vi "nanocal -- nuclear schottky fit V7.vi"() -> ()   [LabVIEW 2021] (continued)
  in  ":sweep is ON":bool
  in  "win":T16={"cen (Hz)"=23772.179970264126, "win (Hz)"=4484.832860239923, "left (Hz)"=21529.763540144166, "right (Hz)"=26014.596400384085}
  in  "cursor window":T17={"left"=20184.313682072192, "right "=24669.14654231211, "center"=22426.730112192152, "window"=4484.832860239923, "cursors"=[0, 1, 2], "relative"=0, "absolute"=0, "fixed vertical offset"=0.0, "vertical offset"=0.0, "skew"=0.0, "default window frac"=0.1, "kind"=enum."symmetric", "skew.left"=0.5, "skew.right"=0.5, "Plot ref"=refnum, "wing order"=enum."forw"}
  out "color data":cluster{"Array":dbl[], "Array":dbl[]}[](array[cluster])=[{"Array"=[0.12, 0.148, 0.15, 0.17, 0.2, 0.25, 0.3, 0.36, 0.42, 0.52, 0.62, 0.82, 1.12, 1.7, 1.9, 3.1, 5.7], "Array"=[0.62728998582, 0.2730109012575849, 0.4360358231158382, 0.31273882707493267, 0.21185679953244455, 0.14497429295634315, 0.10320507255338958, 0.06738649827292763, 0.022507492936216303, 0.021849716434935364, 0.021729475893381252, 0.0198519726342436, 0.016283381951146165, 0.01886089700009046, 0.017534515105553365, 0.01657901647493233, 0.017491792324152208]}, {"Array"=[0.12, 0.148, 0.15, 0.17, 0.2, 0.25, 0.3, 0.36, 0.42, 0.52, 0.62, 0.82, 1.12, 1.7, 1.9, 3.1, 5.7], "Array"=[0.23974349678, 0.07091543775458298, 0.13629832485566626, 0.15316677568416495, 0.17371303124805412, 0.27815367910908206, 0.4568771678095196, 0.03375938315839582, 0.03387143424300576, 0.033883152649051125, 0.03390178634313435, 0.03384656153160249, 0.03390452446017073, 0.03378369231014688, 0.02323861783817173, 0.029207680038740087, 0.02587551529326107]}, {"Array"=[0.12, 0.148, 0.15, 0.17, 0.2, 0.25, 0.3, 0.36, 0.42, 0.52, 0.62, 0.82, 1.12, 1.7, 1.9, 3.1, 5.7], "Array"=[0.076926495749, 0.13557684408337248, 0.03542880244691447, 0.02942840377205427, 0.02504707721851352, 0.020087180736490247, 0.018190810679879554, 0.0163524675075112, 0.016835987172777216, 0.01819702773822382, 0.020153498516221252, 0.023547995635674095, 0.031661688913314306, 0.03349591654527996, 0.014265591932458873, 0.009191722708188048, 0.005854448603805341]}, {"Array"=[0.12, 0.148, 0.15, 0.17, 0.2, 0.25, 0.3, 0.36, 0.42, 0.52, 0.62, 0.82, 1.12, 1.7, 1.9, 3.1, 5.7], "Array"=[0.159415903746, 0.04012911681217574, 0.042141009445427945, 0.032059842594624494, 0.02279985029361622, 0.018878235168909133, 0.020353539568818982, 5.5602042137039274e-05, 0.00021346840235837033, 0.00021340250099372794, 0.00021321792059620005, 0.00027413175252649695, 0.0002745370162211529, 0.0004261574975821111, 0.000383027800546881, 0.0002822141564676873, 0.00033678261197217014]}, {"Array"=[0.12, 0.148, 0.15, 0.17, 0.2, 0.25, 0.3, 0.36, 0.42, 0.52, 0.62, 0.82, 1.12, 1.7, 1.9, 3.1, 5.7], "Array"=[0.000763641667, 0.0009923872987074498, 0.0008634344957269274, 0.000966119229084584, 0.0011194877919145127, 0.0013606502621125451, 0.0015326336783234693, 0.002052818741953473, 0.0017781658353584764, 0.001801850307392029, 0.0018089734240976446, 0.002984103948241005, 0.003250738484609814, 0.0031602960429135524, 0.002949269667352954, 0.002421267656945163, 0.002022629565026247]}, {"Array"=[0.12, 0.148, 0.15, 0.17, 0.2, 0.25, 0.3, 0.36, 0.42, 0.52, 0.62, 0.82, 1.12, 1.7, 1.9, 3.1, 5.7], "Array"=[4.35e-10, 6.439381253023805e-10, 6.308810838918409e-10, 7.625114350763984e-10, 8.195852207774218e-10, 1.2510608054547487e-09, 1.5572561005318226e-09, 2.053450896656566e-09, 2.479707154238972e-09, 3.1313474594286157e-09, 3.806148532350378e-09, 5.213755545903577e-09, 7.2628137959888106e-09, 1.1406421503525573e-08, 1.2895431292182517e-08, 2.227660928974633e-08, 5.4777678949124484e-08]}, {"Array"=[0.12, 0.148, 0.15, 0.17, 0.2, 0.25, 0.3, 0.36, 0.42, 0.52, 0.62, 0.82, 1.12, 1.7, 1.9, 3.1, 5.7], "Array"=[0.245568364347, 0.0645900574929368, 0.08004705050622966, 0.19487148720579237, 0.03351434142711687, 0.02184431417017586, 0.032347659490051216, 0.002480419109659059, 0.007814821925534395, 0.00520013588180238, 0.006296094438005391, 0.001908169809423058, 0.002257620140211018, 0.008605835968785608, 0.0024989962580555026, 0.003215464238537897, 0.003570816055454911]}, {"Array"=[0.12, 0.148, 0.15, 0.17, 0.2, 0.25, 0.3, 0.36, 0.42, 0.52, 0.62, 0.82, 1.12, 1.7, 1.9, 3.1, 5.7], "Array"=[0.022170590915, 0.01641248298202389, 0.002312030386804106, 0.0014819318949486784, 0.00035662888776441895, 0.00015894172062156444, 0.00010225804136915292, 0.0001282920284827463, 0.0003857404741353476, 0.00019678175234393364, 0.0002692480741424916, 0.00013393087590862188, 0.00016283980709594313, 0.00045778261364612133, 0.0003120318371061343, 8.8801730217525e-05, 7.291236500401702e-05]}, {"Array"=[0.12, 0.148, 0.15, 0.17, 0.2, 0.25, 0.3, 0.36, 0.42, 0.52, 0.62, 0.82, 1.12, 1.7, 1.9, 3.1, 5.7], "Array"=[0.126655465898, 0.016122106455977173, 0.019370507574418105, 0.032515587695104, 0.003953255270019443, 0.0013746091281296251, 0.0011727018719404464, 1.3396144617265272e-06, 1.8309382419984372e-05, 1.6694885155659994e-05, 1.6264646942714422e-05, 2.638451785235589e-06, 9.699549898748168e-06, 7.027190427402306e-05, 9.499625775806485e-06, 1.529926658584193e-05, 2.3576375004937536e-05]}]
  out "R(ω) fit out":cdb[](array[numeric])
  in  "parameter map":map{T2, dbl}(c390)
  out "filesnames lookup":map{i32, string}(c390)={0="IDS0183_210310_RAW_cal__sam_", 1="IDS0311_210901_RAW_cal__sam_", 2="IDS0359_210907_RAW_cal__sam_", 3="IDS0412_220525_RAW_cal__sam_", 4="IDS0431_220527_RAW_cal__sam_", 5="IDS0442_220528_RAW_cal__sam_", 6="IDS0464_220530_RAW_cal__sam_", 7="IDS0486_220602_RAW_cal__sam_", 8="IDS0336_210904_RAW_cal__sam_", 9="IDS0346_210904_RAW_cal__sam_", 10="IDS0378_210909_RAW_cal__sam_", 11="IDS0158_210310_RAW_cal__sam_", 12="IDS0300_210427_RAW_cal__sam_", 13="IDS0184_210310_RAW_cal__sam_", 14="IDS0210_210310_RAW_cal__sam_", 15="IDS0379_210909_RAW_cal__sam_", 16="IDS0360_210907_RAW_cal__sam_", 17="IDS0411_220525_RAW_cal__sam_", 18="IDS0427_220526_RAW_cal__sam_", 19="IDS0443_220528_RAW_cal__sam_", 20="IDS0463_220530_RAW_cal__sam_", 21="IDS0487_220602_RAW_cal__sam_", 22="IDS0310_210901_RAW_cal__sam_", 23="IDS0337_210904_RAW_cal__sam_", 24="IDS0347_210906_RAW_cal__sam_", 25="IDS0305_210831_RAW_cal__sam_", 26="IDS0361_210908_RAW_cal__sam_", 27="IDS0380_210909_RAW_cal__sam_", 28="IDS0159_210310_RAW_cal__sam_", 29="IDS0304_210831_RAW_cal__sam_", 30="IDS0312_210901_RAW_cal__sam_", 31="IDS0338_210904_RAW_cal__sam_", 32="IDS0410_220525_RAW_cal__sam_", 33="IDS0432_220527_RAW_cal__sam_", 34="IDS0444_220528_RAW_cal__sam_", 35="IDS0462_220530_RAW_cal__sam_", 36="IDS0485_220601_RAW_cal__sam_", 37="IDS0348_210906_RAW_cal__sam_", 38="IDS0181_210310_RAW_cal__sam_", 39="IDS0424_220526_RAW_cal__sam_", 40="IDS0185_210310_RAW_cal__sam_", 41="IDS0208_210310_RAW_cal__sam_", 42="IDS0209_210310_RAW_cal__sam_", 43="IDS0211_210310_RAW_cal__sam_", 44="IDS0212_210310_RAW_cal__sam_", 45="IDS0213_210310_RAW_cal__sam_", 46="IDS0214_210310_RAW_cal__sam_", 47="IDS0215_210310_RAW_cal__sam_", 48="IDS0216_210310_RAW_cal__sam_", 49="IDS0217_210310_RAW_cal__sam_", 50="IDS0330_210901_RAW_cal__sam_", 51="IDS0331_210901_RAW_cal__sam_", 52="IDS0335_210904_RAW_cal__sam_", 53="IDS0362_210908_RAW_cal__sam_", 54="IDS0377_210909_RAW_cal__sam_", 55="IDS0160_210310_RAW_cal__sam_", 56="IDS0303_210831_RAW_cal__sam_", 57="IDS0313_210901_RAW_cal__sam_", 58="IDS0349_210906_RAW_cal__sam_", 59="IDS0407_220525_RAW_cal__sam_", 60="IDS0441_220527_RAW_cal__sam_", 61="IDS0458_220529_RAW_cal__sam_", 62="IDS0477_220601_RAW_cal__sam_", 63="IDS0161_210310_RAW_cal__sam_", 64="IDS0186_210310_RAW_cal__sam_", 65="IDS0302_210831_RAW_cal__sam_", 66="IDS0363_210908_RAW_cal__sam_", 67="IDS0381_210909_RAW_cal__sam_", 68="IDS0408_220525_RAW_cal__sam_", 69="IDS0425_220526_RAW_cal__sam_", 70="IDS0445_220528_RAW_cal__sam_", 71="IDS0459_220529_RAW_cal__sam_", 72="IDS0478_220601_RAW_cal__sam_", 73="IDS0314_210901_RAW_cal__sam_", 74="IDS0339_210904_RAW_cal__sam_", 75="IDS0350_210906_RAW_cal__sam_", 76="IDS0162_210310_RAW_cal__sam_", 77="IDS0187_210310_RAW_cal__sam_", 78="IDS0301_210831_RAW_cal__sam_", 79="IDS0315_210901_RAW_cal__sam_", 80="IDS0382_210909_RAW_cal__sam_", 81="IDS0409_220525_RAW_cal__sam_", 82="IDS0426_220526_RAW_cal__sam_", 83="IDS0446_220528_RAW_cal__sam_", 84="IDS0460_220529_RAW_cal__sam_", 85="IDS0479_220601_RAW_cal__sam_", 86="IDS0364_210908_RAW_cal__sam_", 87="IDS0340_210904_RAW_cal__sam_", 88="IDS0351_210906_RAW_cal__sam_", 89="IDS0163_210310_RAW_cal__sam_", 90="IDS0188_210310_RAW_cal__sam_", 91="IDS0299_210427_RAW_cal__sam_", 92="IDS0316_210901_RAW_cal__sam_", 93="IDS0341_210904_RAW_cal__sam_", 94="IDS0352_210906_RAW_cal__sam_", 95="IDS0365_210908_RAW_cal__sam_", 96="IDS0383_210910_RAW_cal__sam_", 97="IDS0413_220525_RAW_cal__sam_", 98="IDS0428_220526_RAW_cal__sam_", 99="IDS0447_220528_RAW_cal__sam_", 100="IDS0461_220529_RAW_cal__sam_", 101="IDS0480_220601_RAW_cal__sam_", 102="IDS0164_210310_RAW_cal__sam_", 103="IDS0429_220526_RAW_cal__sam_", 104="IDS0448_220528_RAW_cal__sam_", 105="IDS0481_220601_RAW_cal__sam_", 106="IDS0189_210310_RAW_cal__sam_", 107="IDS0298_210427_RAW_cal__sam_", 108="IDS0317_210901_RAW_cal__sam_", 109="IDS0366_210908_RAW_cal__sam_", 110="IDS0384_210910_RAW_cal__sam_", 111="IDS0414_220525_RAW_cal__sam_", 112="IDS0465_220530_RAW_cal__sam_", 113="IDS0342_210904_RAW_cal__sam_", 114="IDS0353_210906_RAW_cal__sam_", 115="IDS0165_210310_RAW_cal__sam_", 116="IDS0190_210310_RAW_cal__sam_", 117="IDS0430_220526_RAW_cal__sam_", 118="IDS0449_220528_RAW_cal__sam_", 119="IDS0482_220601_RAW_cal__sam_", 120="IDS0297_210427_RAW_cal__sam_", 121="IDS0318_210901_RAW_cal__sam_", 122="IDS0343_210904_RAW_cal__sam_", 123="IDS0354_210906_RAW_cal__sam_", 124="IDS0367_210908_RAW_cal__sam_", 125="IDS0385_210910_RAW_cal__sam_", 126="IDS0415_220525_RAW_cal__sam_", 127="IDS0466_220530_RAW_cal__sam_", 128="IDS0166_210310_RAW_cal__sam_", 129="IDS0191_210310_RAW_cal__sam_", 130="IDS0296_210427_RAW_cal__sam_", 131="IDS0319_210901_RAW_cal__sam_", 132="IDS0344_210904_RAW_cal__sam_", 133="IDS0433_220527_RAW_cal__sam_", 134="IDS0450_220528_RAW_cal__sam_", 135="IDS0467_220530_RAW_cal__sam_", 136="IDS0483_220601_RAW_cal__sam_", 137="IDS0368_210908_RAW_cal__sam_", 138="IDS0386_210910_RAW_cal__sam_", 139="IDS0416_220525_RAW_cal__sam_", 140="IDS0220_210310_RAW_cal__sam_", 141="IDS0167_210310_RAW_cal__sam_", 142="IDS0192_210310_RAW_cal__sam_", 143="IDS0434_220527_RAW_cal__sam_", 144="IDS0451_220528_RAW_cal__sam_", 145="IDS0468_220530_RAW_cal__sam_", 146="IDS0484_220601_RAW_cal__sam_", 147="IDS0295_210427_RAW_cal__sam_", 148="IDS0320_210901_RAW_cal__sam_", 149="IDS0355_210906_RAW_cal__sam_", 150="IDS0369_210908_RAW_cal__sam_", 151="IDS0387_210910_RAW_cal__sam_", 152="IDS0417_220525_RAW_cal__sam_", 153="IDS0168_210310_RAW_cal__sam_", 154="IDS0219_210310_RAW_cal__sam_", 155="IDS0193_210310_RAW_cal__sam_", 156="IDS0418_220525_RAW_cal__sam_", 157="IDS0435_220527_RAW_cal__sam_", 158="IDS0452_220528_RAW_cal__sam_", 159="IDS0469_220530_RAW_cal__sam_", 160="IDS0488_220602_RAW_cal__sam_", 161="IDS0294_210427_RAW_cal__sam_", 162="IDS0321_210901_RAW_cal__sam_", 163="IDS0370_210908_RAW_cal__sam_", 164="IDS0388_210910_RAW_cal__sam_", 165="IDS0169_210310_RAW_cal__sam_", 166="IDS0391_210910_RAW_cal__sam_", 167="IDS0439_220527_RAW_cal__sam_", 168="IDS0395_210910_RAW_cal__sam_", 169="IDS0392_210910_RAW_cal__sam_", 170="IDS0389_210910_RAW_cal__sam_", 171="IDS0218_210310_RAW_cal__sam_", 172="IDS0453_220529_RAW_cal__sam_", 173="IDS0194_210310_RAW_cal__sam_", 174="IDS0293_210427_RAW_cal__sam_", 175="IDS0322_210901_RAW_cal__sam_", 176="IDS0371_210908_RAW_cal__sam_", 177="IDS0390_210910_RAW_cal__sam_", 178="IDS0419_220525_RAW_cal__sam_", 179="IDS0436_220527_RAW_cal__sam_", 180="IDS0454_220529_RAW_cal__sam_", 181="IDS0470_220530_RAW_cal__sam_", 182="IDS0489_220602_RAW_cal__sam_", 183="IDS0170_210310_RAW_cal__sam_", 184="IDS0420_220525_RAW_cal__sam_", 185="IDS0421_220525_RAW_cal__sam_", 186="IDS0471_220530_RAW_cal__sam_", 187="IDS0195_210310_RAW_cal__sam_", 188="IDS0472_220530_RAW_cal__sam_", 189="IDS0306_210831_RAW_cal__sam_", 190="IDS0323_210901_RAW_cal__sam_", 191="IDS0422_220525_RAW_cal__sam_", 192="IDS0437_220527_RAW_cal__sam_", 193="IDS0455_220529_RAW_cal__sam_", 194="IDS0490_220602_RAW_cal__sam_", 195="IDS0372_210908_RAW_cal__sam_", 196="IDS0393_210910_RAW_cal__sam_", 197="IDS0171_210310_RAW_cal__sam_", 198="IDS0196_210310_RAW_cal__sam_", 199="IDS0324_210901_RAW_cal__sam_", 200="IDS0438_220527_RAW_cal__sam_", 201="IDS0456_220529_RAW_cal__sam_", 202="IDS0473_220531_RAW_cal__sam_", 203="IDS0373_210908_RAW_cal__sam_", 204="IDS0394_210910_RAW_cal__sam_", 205="IDS0172_210310_RAW_cal__sam_"}
  out "constrained filename lookup":map{i32, string}(c390)={0="IDS0442_220528_RAW_cal__ref_", 1="IDS0210_210310_RAW_cal__ref_", 2="IDS0443_220528_RAW_cal__ref_", 3="IDS0444_220528_RAW_cal__ref_", 4="IDS0441_220527_RAW_cal__ref_", 5="IDS0445_220528_RAW_cal__ref_", 6="IDS0446_220528_RAW_cal__ref_", 7="IDS0447_220528_RAW_cal__ref_", 8="IDS0448_220528_RAW_cal__ref_", 9="IDS0449_220528_RAW_cal__ref_", 10="IDS0450_220528_RAW_cal__ref_", 11="IDS0451_220528_RAW_cal__ref_", 12="IDS0452_220528_RAW_cal__ref_", 13="IDS0453_220529_RAW_cal__ref_", 14="IDS0454_220529_RAW_cal__ref_", 15="IDS0455_220529_RAW_cal__ref_", 16="IDS0456_220529_RAW_cal__ref_"}
  out "mathematica thing":map{string, map{T2, dbl}}(c390)
  out "temps&degs":map{string, map{T2, dbl}}(c390)
  out "all short filenames":map{string, string}(c390)
  out "all full filenames":map{string, path}(c390)
  out "data file parameters map":map{T2, T18}(c390)
  out "side map to NUM":map{T8, i32}(c390)={enum."sam"=8000, enum."ref"=4000}
  out "side map to STR":map{T8, string}(c390)={enum."sam"="_sam_", enum."ref"="_ref_"}
  out "side map from NUM":map{i32, T8}(c390)={4000=enum."ref", 8000=enum."sam"}
  in  "reverse cursor index map":map{i32, T2}(c390)
  out "state of all selectors":map{T2, map{bool, dbl}}(c390)
  out "state of all selectors string":string="__6.0T__0.0deg__4000side_"
  out "new selector names":map{T2, map{T19, string}}(c390)
  in  "cursor index map":map{T2, i32}(c390)
  in  "load & stuff tab 3":enum32{"Page 2"}(tab)
  in  "load & stuff tab 2":enum32{"Page 2"}(tab)
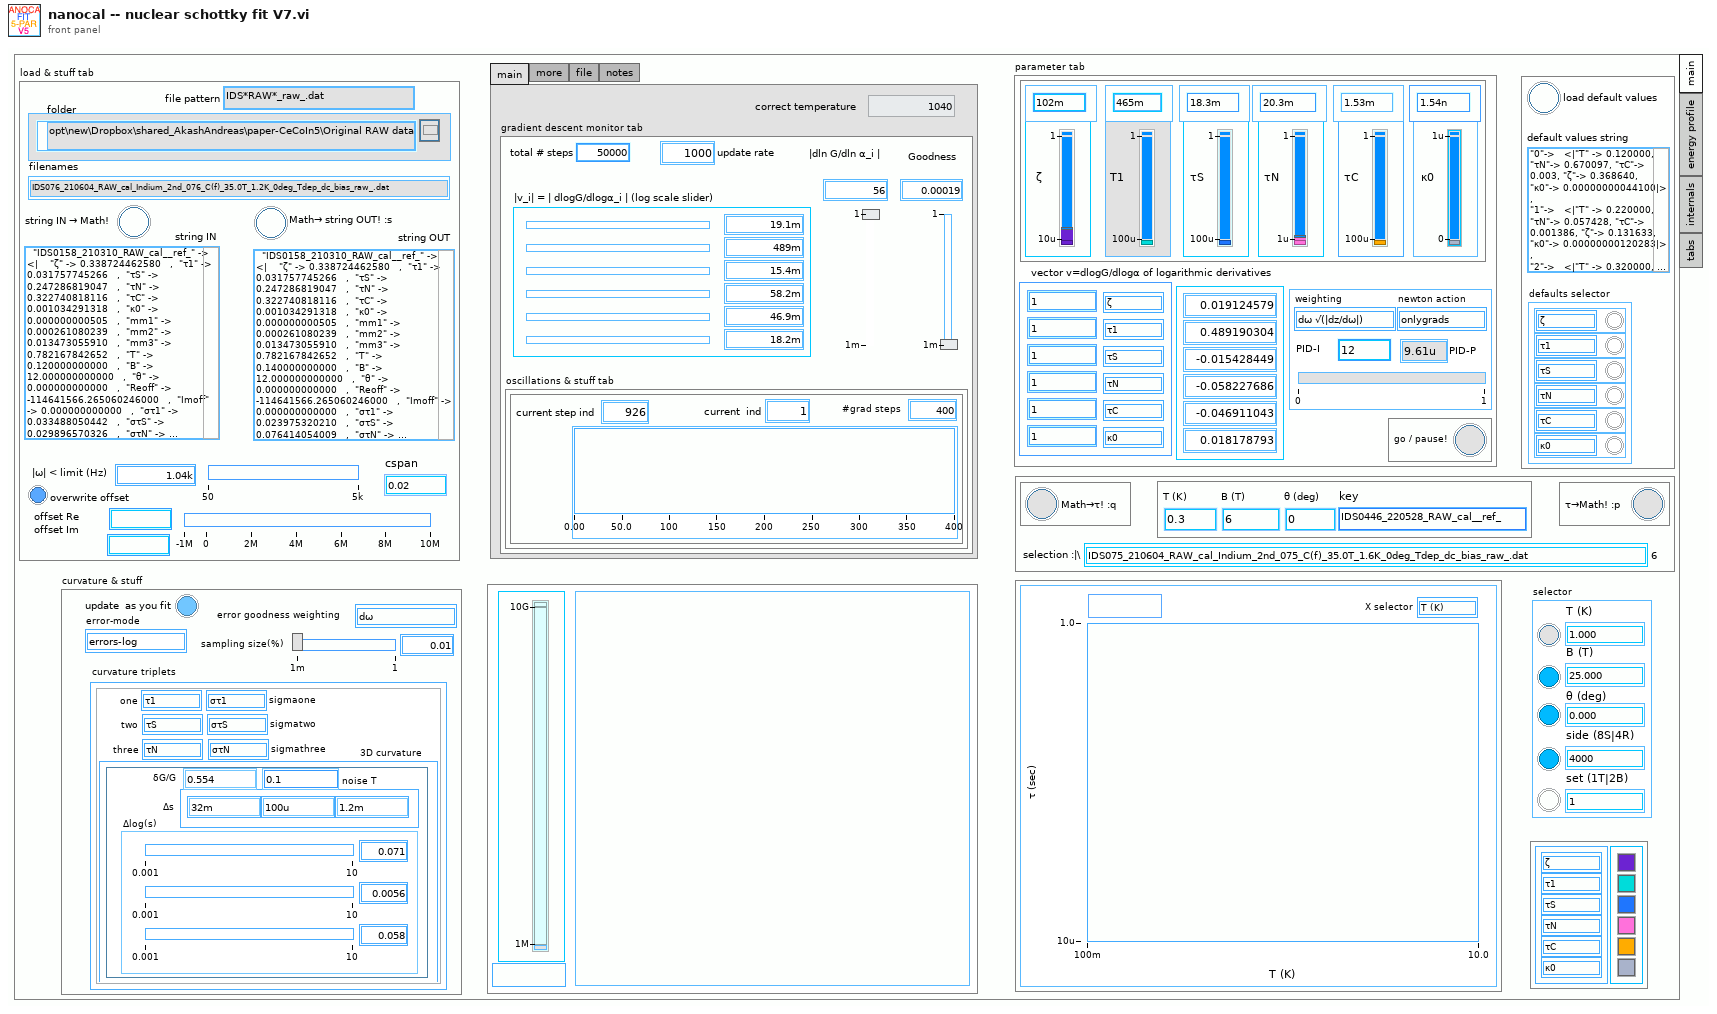
[diagram p1: front panel]
types:
  T1 = enum32{"main", "energy profile", "internals", "tabs"}
  T2 = typedef "3-lorentzian-parameters.ctl" = enum16{"ζ", "τ1", "τS", "τN", "τC", "κ0", "m1", "m2", "m3", "T (K)", "B (T)", "θ (deg)", "side (S|R)", "set of (B|T)", "Re(offset)", "Im(offset)", "στ1", "στ1-", "στ1+", "στS", "στS-", "στS+", "στN", "στN-", "στN+", "τ11", "τ12", "τ21", "τ22", "τN1", "τN2"}
  T3 = typedef "nanocal -- gradient descent -- parameters.ctl" = cluster{"newton action":T4, "weighting":T5, "PID-P":dbl, "PID-I":i32}
  T4 = typedef "3-lorentzian-heat-response action.ctl" = enum16{"calc R", "create string", "calc m1m2m3", "dζ", "dT1", "dτS", "dτN", "dτC", "d-all", "dκ0", "T(K)", "m1", "m2", "m3", "parse string", "θ (deg)", "B (T)", "onlygrads", "newton", "create emty string"}
  T5 = typedef "nanocal-goodness-weighting-strategy.ctl" = enum16{"dω", "dω √(|dz/dω|)", "dω |dz/dω|", "phase", "andreas", "sum", "1/f noise"}
  T6 = typedef "nanocal_data_read_format.ctl" = enum16{"as is", "add - ω", "full rydh", "raw nanocal"}
  T7 = typedef "filename-pattern.ctl" = cluster{"prefix":string, "group":string}
  T8 = typedef "nanocal_side_selector.ctl" = enum16{"sam", "ref"}
  T9 = cluster{"Plost: sweep window":T2, "used default":bool}[]
  T10 = cluster{"ignore set of !":bool, "set (1T|2B)":i32, "ignore side !":bool, "side (8S|4R)":i32, "ignore θ !":bool, "ignore B !":bool, "T (K)":u16, "ignore T !":bool, "θ (deg)":u16, "B (T)":u16, "lookup":cluster{"set of lookup":map{i32, dbl}, "all set of":set{dbl}, "T lookup":map{i32, dbl}, "θ lookup":map{i32, dbl}, "B lookup":map{i32, dbl}, "all T's":set{dbl}, "all θ's":set{dbl}, "all B's":set{dbl}, "all sides":set{dbl}, "side lookup":map{i32, dbl}}}
  T11 = typedef "3D curvature triplet control.ctl" = cluster{"one":T2, "two":T2, "sigmaone":T2, "sigmatwo":T2, "3D curvature":T12, "three":T2, "sigmathree":T2, "pars & errors":map{T2, dbl}}
  T12 = typedef "3D curvature tensor.ctl" = cluster{"curvature Matrix":T13, "eigenvs":dbl[], "Eigenvectors":T14, "theta (rad)":dbl, "theta (deg)":dbl, "Δs":dbl[], "δG/G":dbl, "Δlog(s)":dbl[], "inverse Matrix":T13, "noise T":dbl}
  T13 = typedef "NI_Matrix.lvlib/RealMatrix.ctl" = dbl[][]
  T14 = typedef "NI_Matrix.lvlib/ComplexMatrix.ctl" = cdb[][]
  T15 = typedef "nanocal generate curvature ellipse -- action.ctl" = enum16{"errors-log", "errors-linear"}
  T16 = typedef "show-win- control.ctl" = cluster{"cen (Hz)":dbl, "win (Hz)":dbl, "left (Hz)":dbl, "right (Hz)":dbl}
  T17 = typedef "cursor winow.ctl" = cluster{"left":dbl, "right ":dbl, "center":dbl, "window":dbl, "cursors":i32[], "relative":i32, "absolute":i32, "fixed vertical offset":dbl, "vertical offset":dbl, "skew":dbl, "default window frac":dbl, "kind":enum16{"symmetric", "skewed", "fancy"}, "skew.left":dbl, "skew.right":dbl, "Plot ref":refnum<vi>, "wing order":enum16{"forw", "back"}}
  T18 = typedef "filename-action.ctl" = enum16{"rewrite", "parse", "force pattern", "uniquenum", "get T", "get B", "get ind", "get deg", "get name", "get folder", "get extension", "get basename", "get side", "get setof", "getID", "getIDStock"}
  T19 = typedef "nameformattingitem.ctl" = enum16{"name", "nameL", "units", "prec"}
  T20 = cluster{"keys":T2[], "regexps":string[], "labels":string[]}
  T21 = typedef "cursor action.ctl" = enum16{"range", "read", "write", "check", "zoom out", "smart zoom out", "zoom to aspect ratio 1", "zoom to win", "zoom out 20%", "zoom in 20%", "-empty", "smart zoom out&aspect", "move range left 20%", "move range right 20%", "move range up 20%", "move range down 20%", "zoom to X win", "zoom to Y win", "zoom out X", "zoom out Y", "zoom in X", "zoom in Y", "check plot scale", "set plot color", "set Xlabel", "set Ylabel", "set cursor color"}
  T22 = typedef "cursor window action.ctl" = enum16{"balance", "h. offset change", "cursor moves", "change center", "change window", "init", "check", "reset", "set y to middle", "idle", "-write all Y", "-write left.X", "-write center.X", "-write right.X", "-write all X", "-change center", "-change window", "-change skew", "-read cursor 2", "-read cursor 1", "-read cursor 0", "-read all cursors", "-reset", "-read plot scale", "-set y to middle", "-Q: center.Y is visible", "-Q: window is visible", "-parse center.Y", "-right left from center", "-left move", "-right move", "-set center.Y", "-empty", "-set cursors to default", "-check", "-write center.Y", "-copy cursor 1", "-copy cursor 0", "-copy cursor 2", "move right", "move left", "shrink", "broaden", "skew up", "skew down", "-write plot scale", "zoom X", "change cen&win", "zoom to all data", "color--red", "color--green", "color--yellow", "read", "zoom out", "zoom in", "slide right", "slide left", "set range aspect ratio to 1", "move to window range", "--move to window range"}
  T23 = typedef "publisher action.ctl" = enum16{"set", "get", "init", "check"}
  T24 = typedef "nanocal -- gradient descent -- action.ctl" = enum16{"init", "step", "peek"}
  T25 = typedef "cursor sate.ctl" = enum16{"normal", "alert", "fuzzy", "interesting", "boring", "colored"}
  T26 = typedef "mathematica string map action.ctl" = enum16{"create string", "calc m1m2m3", "parse string"}
  T27 = typedef "LVMapReplaceAction.ctl" = enum32{"Modify Entry only if found", "Add or Modify Entry", "Delete Entry"}
  T28 = typedef "nanocal -- defaut parameter manager action-- V1.ctl" = enum16{"get logarithmic interp", "update", "get linear interp"}
  T29 = typedef "nanocal -- plotstring file action.ctl" = enum16{"generate plotstring file", "generate plotstring thing", ""}
  T30 = typedef "file -- read-write control.ctl" = enum16{"read", "write all", "append one line"}
  T31 = typedef "nanocal_raw_file_manage_action_V1.ctl" = enum16{"read S side", "read R side", "read meta", "read_names"}
  T32 = typedef "array -- freq-voltage transformations action.ctl" = enum16{"as is", "add -ω", "sort ω", "2 x ω", "R-phase(deg) to Re-Im", "select ω>0", "labview file str", "select |ω|<max"}
  T33 = typedef "KM_file -- read-write control.ctl" = enum16{"read", "write all", "append one line"}
  T34 = typedef "nanocal -- gradient descent-- data.ctl" = cluster{"dz/dω  (sec/rad)":cdb[], "z ":cdb[], "ω (rad/sec)":dbl[]}
  T35 = typedef "array action.ctl" = enum16{"generate range", "generate log range"}
  T36 = typedef "LVRangeTypeDef.ctl" = cluster{"Minimum":dbl, "Maximum":dbl, "Increment":dbl, "Minor Increment":dbl, "Start":dbl}
  T37 = typedef "2Dwindow.ctl" = cluster{"window y":dbl, "center x":dbl, "center y":dbl, "window x":dbl}
  T38 = typedef "eventvkey.ctl" = enum16{"ASCII", "Enter", "Return", "Shift", "Ctrl", "Alt", "Cmd", "Opt", "Caps", "NumLock", "Clear", "Break", "Up", "Down", "Left", "Right", "Insert", "Delete", "Home", "End", "PageUp", "PageDown", "Escape", "Help", "Pause", "ScrollLock", "F1", "F2", "F3", "F4", "F5", "F6", "F7", "F8", "F9", "F10", "F11", "F12", "F13", "F14", "F15", "F16", "F17", "F18", "F19", "F20", "F21", "F22", "F23", "F24", "Play", "VolumeUp", "VolumeDown", "Mute", "Two Byte Char"}
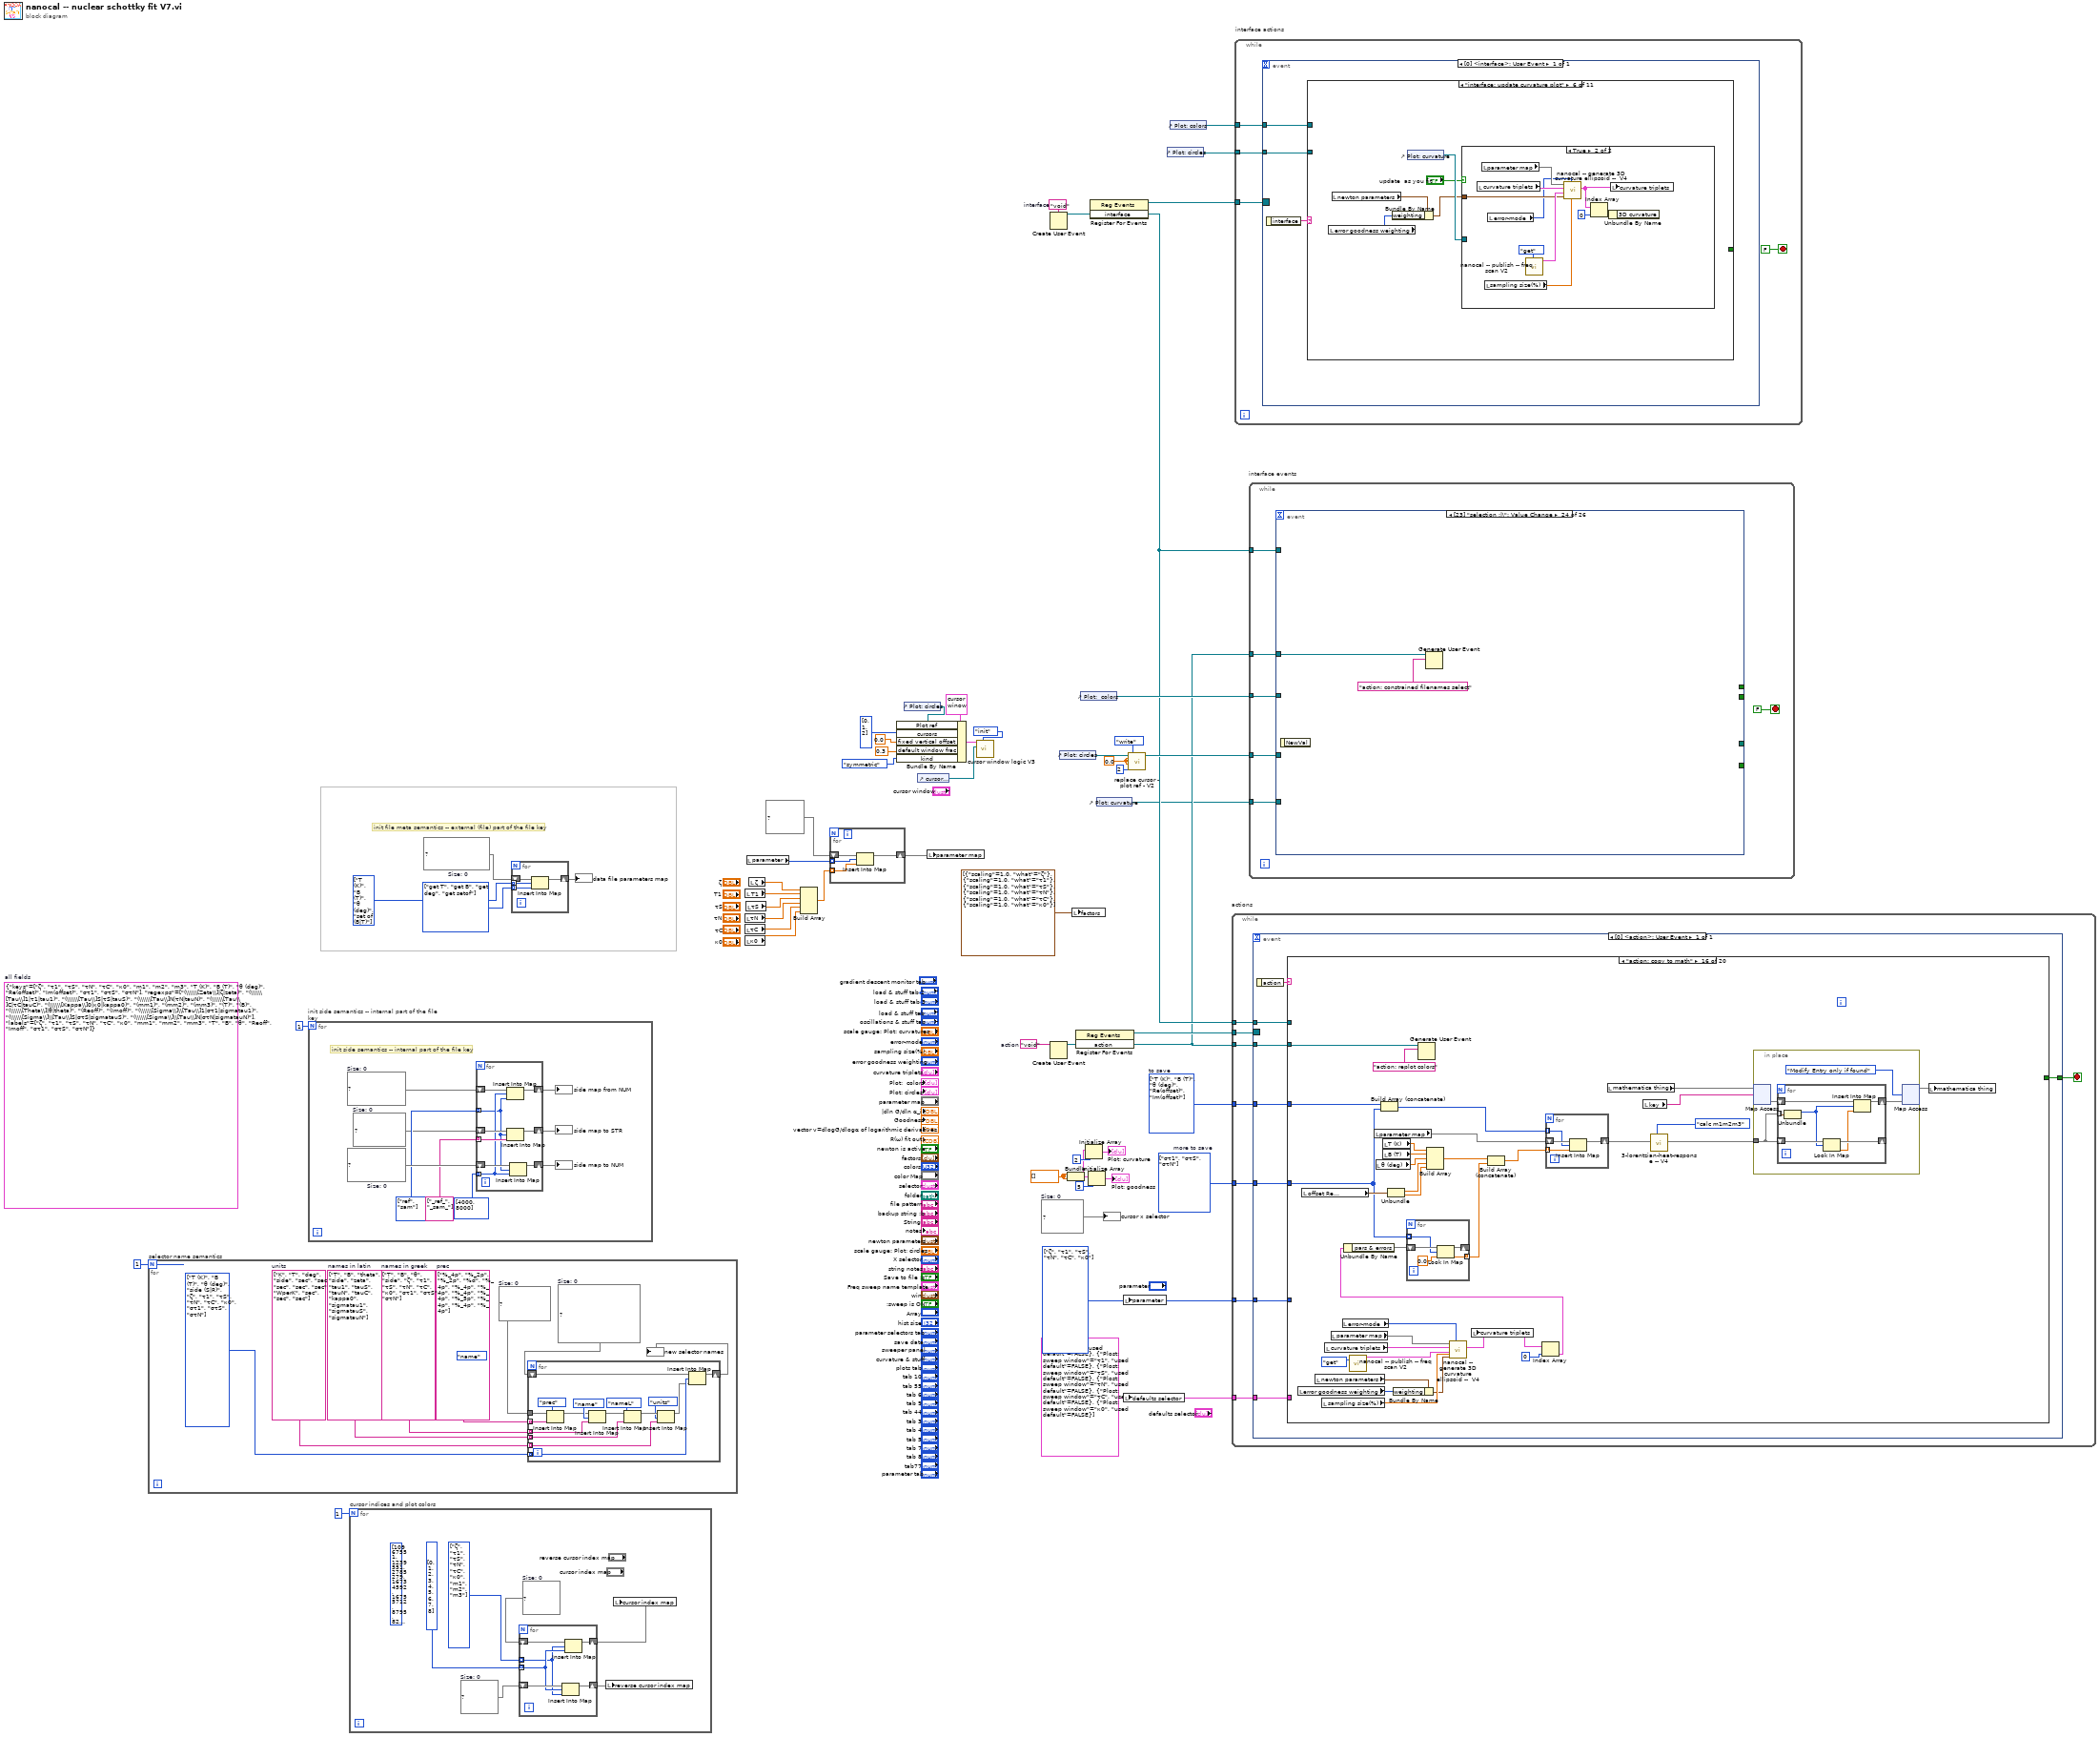
[diagram p0: block diagram]
diagram:
  w1 = T2[] [enum."T (K)", enum."B (T)", enum."θ (deg)", enum."Re(offset)", enum."Im(offset)"] items=["ζ", "τ1", "τS", "τN", "τC", "κ0", "m1", "m2", "m3", "T (K)", "B (T)", "θ (deg)", "side (S|R)", "set of (B|T)", "Re(offset)", "Im(offset)", "στ1", "στ1-", "στ1+", "στS", "στS-", "στS+", "στN", "στN-", "στN+", "τ11", "τ12", "τ21", "τ22", "τN1", "τN2"]  # to save
  w2 = T2[] [enum."στ1", enum."στS", enum."στN"] items=["ζ", "τ1", "τS", "τN", "τC", "κ0", "m1", "m2", "m3", "T (K)", "B (T)", "θ (deg)", "side (S|R)", "set of (B|T)", "Re(offset)", "Im(offset)", "στ1", "στ1-", "στ1+", "στS", "στS-", "στS+", "στN", "στN-", "στN+", "τ11", "τ12", "τ21", "τ22", "τN1", "τN2"]  # more to save
  (unwired) T20 {"keys"=[enum."ζ", enum."τ1", enum."τS", enum."τN", enum."τC", enum."κ0", enum."m1", enum."m2", enum."m3", enum."T (K)", enum."B (T)", enum."θ (deg)", enum."Re(offset)", enum."Im(offset)", enum."στ1", enum."στS", enum."στN"], "regexps"=["(\\\\\\[Zeta\\]|ζ|zeta)", "(\\\\\\[Tau\\]1|τ1|tau1)", "(\\\\\\[Tau\\]S|τS|tauS)", "(\\\\\\[Tau\\]N|τN|tauN)", "(\\\\\\[Tau\\]C|τC|tauC)", "(\\\\\\[Kappa\\]0|κ0|kappa0)", "(mm1)", "(mm2)", "(mm3)", "(T)", "(B)", "(\\\\\\[Theta\\]|θ|theta)", "(Reoff)", "(Imoff)", "(\\\\\\[Sigma\\]\\[Tau\\]1|στ1|sigmatau1)", "(\\\\\\[Sigma\\]\\[Tau\\]S|στS|sigmatauS)", "(\\\\\\[Sigma\\]\\[Tau\\]N|στN|sigmatauN)"], "labels"=["ζ", "τ1", "τS", "τN", "τC", "κ0", "mm1", "mm2", "mm3", "T", "B", "θ", "Reoff", "Imoff", "στ1", "στS", "στN"]}  # all fields
  w26 = T9 [{"Plost: sweep window"=enum."ζ", "used default"=FALSE}, {"Plost: sweep window"=enum."τ1", "used default"=FALSE}, {"Plost: sweep window"=enum."τS", "used default"=FALSE}, {"Plost: sweep window"=enum."τN", "used default"=FALSE}, {"Plost: sweep window"=enum."τC", "used default"=FALSE}, {"Plost: sweep window"=enum."κ0", "used default"=FALSE}] ("parameter 2")
  w27 = T18[] [enum."get T", enum."get B", enum."get deg", enum."get setof"] items=["rewrite", "parse", "force pattern", "uniquenum", "get T", "get B", "get ind", "get deg", "get name", "get folder", "get extension", "get basename", "get side", "get setof", "getID", "getIDStock"]
  w29 = map{T2, T18} {}  # Size: 0
  w28 = T2[] [enum."T (K)", enum."B (T)", enum."θ (deg)", enum."set of (B|T)"] items=["ζ", "τ1", "τS", "τN", "τC", "κ0", "m1", "m2", "m3", "T (K)", "B (T)", "θ (deg)", "side (S|R)", "set of (B|T)", "Re(offset)", "Im(offset)", "στ1", "στ1-", "στ1+", "στS", "στS-", "στS+", "στN", "στN-", "στN+", "τ11", "τ12", "τ21", "τ22", "τN1", "τN2"]
  w33 = dbl[] []
  w22 = T2[] [enum."ζ", enum."τ1", enum."τS", enum."τN", enum."τC", enum."κ0"] items=["ζ", "τ1", "τS", "τN", "τC", "κ0", "m1", "m2", "m3", "T (K)", "B (T)", "θ (deg)", "side (S|R)", "set of (B|T)", "Re(offset)", "Im(offset)", "στ1", "στ1-", "στ1+", "στS", "στS-", "στS+", "στN", "στN-", "στN+", "τ11", "τ12", "τ21", "τ22", "τN1", "τN2"]
  w36 = map{T2, dbl} {}  # Size: 0
  w37 = 0.0 ("new X")
  w50 = "void"  # interface
  w51 = "void"  # action
  # "init file meta semantics -- external (file) part of the file key"
  n1 = for "selector name semantics" {
    N: 1 -> [_]
    w53 = string[] ["%_4p", "%_2p", "%_2p", "%d", "%_4p", "%_4p", "%_4p", "%_4p", "%_4p", "%_5p", "%_4p", "%_4p", "%_4p"]  # prec
    w57 = map{T19, string} {}  # Size: 0
    (unwired) nameformattingitem."name" ("name formatting item")
    w55 = string[] ["K", "T", "deg", "side", "sec", "sec", "sec", "sec", "sec", "WperK", "sec", "sec", "sec"]  # units
    w58 = string[] ["T", "B", "theta", "side", "zeta", "tau1", "tauS", "tauN", "tauC", "kappa0", "sigmatau1", "sigmatauS", "sigmatauN"]  # names in latin
    w56 = string[] ["T", "B", "θ", "side", "ζ", "τ1", "τS", "τN", "τC", "κ0", "στ1", "στS", "στN"]  # names in greek
    w60 = map{T2, map{T19, string}} {}  # Size: 0
    w59 = T2[] [enum."T (K)", enum."B (T)", enum."θ (deg)", enum."side (S|R)", enum."ζ", enum."τ1", enum."τS", enum."τN", enum."τC", enum."κ0", enum."στ1", enum."στS", enum."στN"] items=["ζ", "τ1", "τS", "τN", "τC", "κ0", "m1", "m2", "m3", "T (K)", "B (T)", "θ (deg)", "side (S|R)", "set of (B|T)", "Re(offset)", "Im(offset)", "στ1", "στ1-", "στ1+", "στS", "στS-", "στS+", "στN", "στN-", "στN+", "τ11", "τ12", "τ21", "τ22", "τN1", "τN2"]
    n2 = for {
      shift-right: [w75] -> w54
      shift-left: w60 -> [w76]
      tunnel: w58 -> [w66] mode=indexing
      tunnel: w59 -> [w74] mode=indexing
      tunnel: w57 -> [w64]
      tunnel: w56 -> [w65] mode=indexing
      tunnel: w55 -> [w67] mode=indexing
      tunnel: w53 -> [w63] mode=indexing
      n3 = Insert Into Map(map in=w64, key=nameformattingitem."prec", value=w63) -> (map out=w62:map{T19, string})  [unwired: 2 out]
      n4 = Insert Into Map(map in=w62, key=nameformattingitem."name", value=w65) -> (map out=w73:map{T19, string})  [unwired: 2 out]
      n5 = Insert Into Map(map in=w73, key=nameformattingitem."nameL" ("name formatting item"), value=w66) -> (map out=w72:map{T19, string})  [unwired: 2 out]
      n6 = Insert Into Map(map in=w72, key=nameformattingitem."units" ("name formatting item"), value=w67) -> (map out=w71:map{T19, string})  [unwired: 2 out]
      n7 = Insert Into Map(map in=w76, key=w74, value=w71) -> (map out=w75:map{T2, map{T19, string}})  [unwired: 2 out]
    }
    "new selector names" <- w54
  }
  n8 = for "init side semantics -- internal part of the file key" {
    N: 1 -> [_]
    w78 = map{i32, T8} {}  # Size: 0
    w80 = map{T8, string} {}  # Size: 0
    w81 = T8[] [enum."ref", enum."sam"] items=["sam", "ref"]
    w85 = map{T8, i32} {}  # Size: 0
    # "init side semantics -- internal part of the file key"
    n9 = for {
      shift-right: [w93] -> w82
      shift-left: w85 -> [w94]
      tunnel: string[] ["_ref_", "_sam_"] -> [w90] mode=indexing
      tunnel: i32[] [4000, 8000] -> [w87] mode=indexing
      tunnel: w81 -> [w86] mode=indexing
      shift-right: [w91] -> w79
      shift-left: w80 -> [w92]
      shift-right: [w88] -> w77
      shift-left: w78 -> [w89]
      n10 = Insert Into Map(map in=w89, key=w87, value=w86) -> (map out=w88:map{i32, T8})  [unwired: 2 out]
      n11 = Insert Into Map(map in=w92, key=w86, value=w90) -> (map out=w91:map{T8, string})  [unwired: 2 out]
      n12 = Insert Into Map(map in=w94, key=w86, value=w87) -> (map out=w93:map{T8, i32})  [unwired: 2 out]
    }
    "side map from NUM" <- w77
    "side map to STR" <- w79
    "side map to NUM" <- w82
  }
  n13 = for "cursor indices and plot colors" {
    N: 1 -> [_]
    w96 = map{i32, T2} {}  # Size: 0
    (unwired) u32[] [10967551, 1239551, 2785279, 16734592, 16755712, 8795, 8285330, 9272482, 9204890]
    w100 = map{T2, i32} {}  # Size: 0
    w97 = T2[] [enum."ζ", enum."τ1", enum."τS", enum."τN", enum."τC", enum."κ0", enum."m1", enum."m2", enum."m3"] items=["ζ", "τ1", "τS", "τN", "τC", "κ0", "m1", "m2", "m3", "T (K)", "B (T)", "θ (deg)", "side (S|R)", "set of (B|T)", "Re(offset)", "Im(offset)", "στ1", "στ1-", "στ1+", "στS", "στS-", "στS+", "στN", "στN-", "στN+", "τ11", "τ12", "τ21", "τ22", "τN1", "τN2"]
    n14 = for {
      shift-right: [w105] -> w98
      shift-left: w100 -> [w106]
      tunnel: w97 -> [w101] mode=indexing
      tunnel: i32[] [0, 1, 2, 3, 4, 5, 6, 7, 8] -> [w102] mode=indexing
      shift-right: [w103] -> w95
      shift-left: w96 -> [w104]
      n15 = Insert Into Map(map in=w104, key=w102, value=w101) -> (map out=w103:map{i32, T2})  [unwired: 2 out]
      n16 = Insert Into Map(map in=w106, key=w101, value=w102) -> (map out=w105:map{T2, i32})  [unwired: 2 out]
    }
    n17 = local write "reverse cursor index map"(w95) -> ()
    n18 = local write "cursor index map"(w98) -> ()
  }
  n19 = for {
    shift-right: [w109] -> w30
    shift-left: w29 -> [w110]
    tunnel: w28 -> [w108] mode=indexing
    tunnel: w27 -> [w107] mode=indexing
    n20 = Insert Into Map(map in=w110, key=w108, value=w107) -> (map out=w109:map{T2, T18})  [unwired: 2 out]
  }
  "data file parameters map" <- w30
  n21 = local read "τN"() -> (w16:dbl)
  n22 = local read "τC"() -> (w17:dbl)
  n23 = local read "κ0"() -> (w18:dbl)
  n24 = local read "T1"() -> (w14:dbl)
  n25 = local read "τS"() -> (w15:dbl)
  n26 = local read "parameter"() -> (w20:T2[])
  n27 = local read "ζ"() -> (w13:dbl)
  n28 = Build Array(w13, w14, w15, w16, w17, w18) -> (w19:dbl[])
  n29 = for {
    shift-right: [w113] -> w21
    shift-left: map{T2, dbl} {} ("Map IN") -> [w114]
    tunnel: w20 -> [w112] mode=indexing
    tunnel: w19 -> [w111] mode=indexing
    n30 = Insert Into Map(map in=w114, key=w112, value=w111) -> (map out=w113:map{T2, dbl})  [unwired: 2 out]
  }
  n31 = control-ref of="Plot: circles"() -> (w42:refnum<vi>)
  n32 = Bundle By Name(cluster=T17 {"left"=0.0, "right "=0.0, "center"=0.0, "window"=0.0, "cursors"=[], "relative"=0, "absolute"=0, "fixed vertical offset"=0.0, "vertical offset"=0.0, "skew"=0.0, "default window frac"=0.0, "kind"=enum."symmetric", "skew.left"=0.0, "skew.right"=0.0, "Plot ref"=refnum, "wing order"=enum."forw"} ("cursor bracket: All, data window"), "Plot ref"=w42, "cursors"=i32[] [0, 1, 2], "fixed vertical offset"=0.0, "default window frac"=0.3 ("fixed vertical offset"), "kind"=enum16{"symmetric", "skewed", "fancy"}."symmetric") -> (w45:T17)
  n33 = control-ref of="cursor window"() -> (w41:refnum<vi>)
  n34 = local write "parameter map"(w21) -> ()
  n35 = call "cursor window logic V3.vi"("cursor window action"=cursor_window_action."init", "cursor window in"=w41, "cursor window init"=w45) -> ()  [unwired: 7 in, 2 out]
  n36 = Create User Event(user event datatype=w50) -> (user event=w10:refnum<user-event>)  [unwired: 1 in, 1 out]
  n37 = Create User Event(user event datatype=w51) -> (user event=w9:refnum<user-event>)  [unwired: 1 in, 1 out]
  n38 = control-ref of="Plot: circles"() -> (w38:refnum<vi>)
  n39 = Bundle(w33, w33) -> (w5:cluster{dbl[], dbl[]})  [unwired: 1 in]
  n40 = local write "factors"(cluster{"scaling":dbl, "what":T2}[] [{"scaling"=1.0, "what"=enum."ζ"}, {"scaling"=1.0, "what"=enum."τ1"}, {"scaling"=1.0, "what"=enum."τS"}, {"scaling"=1.0, "what"=enum."τN"}, {"scaling"=1.0, "what"=enum."τC"}, {"scaling"=1.0, "what"=enum."κ0"}]) -> ()
  n41 = register-events(w9) -> (reference out=w52:refnum<event-registration>)  [unwired: 2 in, 1 out]
  n42 = control-ref of="Plot:  colors"() -> (w35:refnum<vi>)
  n43 = Initialize Array(w5, 2 ("dimension size")) -> (→"Plot: curvature":cluster{dbl[], dbl[]}[])
  n44 = Initialize Array(w5, 5 ("dimension size")) -> (→"Plot: goodness":cluster{dbl[], dbl[]}[])
  n45 = register-events(w10) -> (reference out=w11:refnum<event-registration>)  [unwired: 2 in, 1 out]
  n46 = control-ref of="Plot: curvature"() -> (w3:refnum<vi>)
  n47 = local write "parameter"(w22) -> ()
  n48 = local write "defaults selector"(w26) -> ()
  n49 = call "replace cursor - plot ref - V2.vi"("Plot ref in"=w38, "new X"=w37, "new  Y"=w37, "cursor index"=2, "cursor action"=cursor_action."write") -> ()  [unwired: 11 in, 4 out]
  n50 = control-ref of="Plot: circles"() -> (w7:refnum<vi>)
  n51 = control-ref of="Plot: colors"() -> (w8:refnum<vi>)
  n52 = while "actions" {
    tunnel: w52 -> [w122]
    tunnel: w9 -> [w121]
    tunnel: w10 -> [w119]
    tunnel: w22 -> [w118]
    tunnel: w26 -> [w117]
    tunnel: w2 -> [w116]
    tunnel: w1 -> [w115]
    stop <- w120 stop-if-true
    n53 = event shown="[0] <action>: User Event" {
      selector: w122 -> [_]
      dyn-events: _ -> [_]
      timeout: _ -> [_]
      tunnel: w121 -> [w129]
      tunnel: [w128] -> w120
      tunnel: w119 -> [w127]
      tunnel: w118 -> [w126]
      tunnel: w117 -> [w125]
      tunnel: w116 -> [w124]
      tunnel: w115 -> [w123]
      event User Event {
        n54 = event-data() -> ("action"=w130:string)  [unwired: 1 in]
        n55 = case shown="\"action: copy to math\"" w130 {
          tunnel: w129 -> [w138 _ _ _ w321 w346 _ _ w539 _ w666 _ _ w772 w824 w925 _ w987 _ _]
          tunnel: [_ _ _ _ _ _ _ _ _ _ _ _ _ _ _ _ TRUE _ _ _] -> w128
          tunnel: w127 -> [w141 w145 _ w266 w315 _ _ _ _ _ _ _ w682 _ w814 _ _ _ _ _]
          tunnel: w126 -> [_ w152 w161 w265 _ _ w473 _ _ _ _ _ w680 _ w820 _ _ _ _ _]
          tunnel: w125 -> [_ _ _ _ _ _ _ _ _ _ _ _ _ _ _ _ _ _ _ _]
          tunnel: w124 -> [_ _ _ _ _ _ _ _ _ _ _ _ w678 _ _ w896 _ _ _ _]
          tunnel: w123 -> [_ _ _ _ _ _ _ _ _ _ _ _ _ _ _ w893 _ _ _ _]
          frame "action: new sweep" {
            n56 = Generate User Event(user event=w141, event data cluster="interface: update plot colors cursors" ("event data")) -> (user event out=w142:refnum<user-event>)  [unwired: 2 in, 1 out]
            n57 = Generate User Event(user event=w142, event data cluster="interface: reset colors" ("event data")) -> ()  [unwired: 2 in, 2 out]
            n58 = Generate User Event(user event=w138, event data cluster="action: replot circles" ("event data")) -> ()  [unwired: 2 in, 2 out]
            n59 = call "nanocal -- publish -- freq scan V2.vi"("publisher action"=publisher_action."get") -> ("z out (V)"=w137:cdb[])  [unwired: 7 in, 3 out]
            n60 = control-ref of="Plot: circles"() -> (w132:refnum<vi>)
            n61 = Complex To Re/Im(x + iy=w137) -> (x=w135:dbl[], y=w136:dbl[])
            n62 = call "replace plot - plot ref - V2.vi"("Plot ref in"=w132, "Array X IN"=w135, "Array Y IN"=w136, "plot index"=enum16{"data R(ω)", "fit R(ω)"}."data R(ω)" ("Plost: sweep window"), "cursor action"=cursor_action."write") -> ()  [unwired: 11 in, 4 out]
          }
          frame "action: replot circles" {
            n63 = local read "newton parameters"() -> (w153:T3)
            n64 = local read "parameter map"() -> (w147:map{T2, dbl})
            n65 = call "nanocal -- publish -- freq scan V2.vi"("publisher action"=publisher_action."get") -> ("data"=w151:T34)  [unwired: 7 in, 3 out]
            n66 = call "nanocal -- gradient descent.vi"("data"=w151, "action"=nanocal_--_gradient_descent_--_action."peek", "newton pars"=w153, "parameter keys IN"=w152, "parameter Map IN"=w147) -> ("logarithmic derivatives OUT"=w148:dbl[], "R(ω) out"=w146:cdb[], "goodness OUT"=w150:dbl)  [unwired: 2 in, 2 out]
            n67 = local write "vector v=dlogG/dlogα of logarithmic derivatives"(w148) -> ()
            n68 = Absolute Value(x=w148) -> (abs(x)=w149:dbl[])
            n69 = flat-sequence {
              tunnel: w146 -> [w156]
              tunnel: w145 -> [w158]
              tunnel: "interface: update circle fit plot" ("event data") -> [w157]
              frame #0 {
                n70 = local write "R(ω) fit out"(w156) -> ()
              }
              frame #1 {
                n71 = Generate User Event(user event=w158, event data cluster=w157) -> ()  [unwired: 2 in, 2 out]
              }
            }
            n72 = local write "Goodness"(w150) -> ()
            n73 = local write "|v_i| = | dlogG/dlogα_i | (log scale slider)"(w149) -> ()
          }
          frame "action: plot landscape" {
            w172 = array_action."generate log range" ("action")
            n74 = property on="range one" class="Slide (strict)"() -> ("Scale.Range"=w181:T36)  [unwired: 2 in, 2 out]
            n75 = property on="range two" class="Slide (strict)"() -> ("Scale.Range"=w180:T36)  [unwired: 2 in, 2 out]
            n76 = Unbundle By Name(w181) -> ("Maximum"=w175:dbl, "Minimum"=w174:dbl)
            n77 = Unbundle By Name(w180) -> ("Maximum"=w177:dbl, "Minimum"=w176:dbl)
            n78 = local read "cursor index map"() -> (w167:map{T2, i32})
            n79 = call "array -- generate range -- V5.vi"("action"=w172, "ω points"="# points", "ω from"=w176, "ω to"=w177) -> ("ω out"=w178:dbl[])  [unwired: 7 in]
            n80 = local read "color Map"() -> (w168:map{T2, u32})
            n81 = call "array -- generate range -- V5.vi"("action"=w172, "ω points"="# points", "ω from"=w174, "ω to"=w175) -> ("ω out"=w173:dbl[])  [unwired: 7 in]
            n82 = call "nanocal -- publish -- freq scan V2.vi"("publisher action"=publisher_action."get") -> ("data"=w160:T34)  [unwired: 7 in, 3 out]
            n83 = local read "newton parameters"() -> (w162:T3)
            n84 = local read "parameter map"() -> (w159:map{T2, dbl})
            n85 = Look In Map(map=w168, key="two") -> (value=w170:u32)  [unwired: 1 in, 1 out]
            n86 = Look In Map(map=w168, key="one") -> (value=w169:u32)  [unwired: 1 in, 1 out]
            n87 = Build Array("one", "two") -> (w166:T2[])
            n88 = property on="range one" class="Slide (strict)"("Fill Color"=w169) -> ()  [unwired: 2 in, 2 out]
            n89 = property on="range two" class="Slide (strict)"("Fill Color"=w170) -> ()  [unwired: 2 in, 2 out]
            n90 = case shown="\"1d plots\", Default" "what" {
              tunnel: w159 -> [w189 w229]
              tunnel: "one" -> [_ w228]
              tunnel: w178 -> [_ w227]
              tunnel: w173 -> [w188 w226]
              tunnel: "two" -> [_ w225]
              tunnel: w168 -> [w187 _]
              tunnel: w167 -> [w186 _]
              tunnel: w166 -> [w183 _]
              tunnel: w160 -> [w184 w220]
              tunnel: w162 -> [w182 w218]
              tunnel: w161 -> [_ w219]
              frame "1d plots", Default {
                n91 = control-ref of="Plot: goodness"() -> (w185:refnum<vi>)
                n92 = for {
                  tunnel: w189 -> [w196]
                  tunnel: w188 -> [w205]
                  tunnel: w183 -> [w195] mode=indexing
                  tunnel: w187 -> [w202]
                  tunnel: w186 -> [w201]
                  tunnel: w185 -> [w193]
                  tunnel: w184 -> [w192]
                  tunnel: w183 -> [w191]
                  tunnel: w182 -> [w190]
                  n93 = for {
                    tunnel: w205 -> [w209] mode=indexing
                    tunnel: [w210] -> w207 mode=indexing
                    tunnel: [w209] -> w206 mode=indexing
                    tunnel: w196 -> [w216]
                    tunnel: w195 -> [w217]
                    tunnel: w192 -> [w215]
                    tunnel: w191 -> [w212]
                    tunnel: w190 -> [w211]
                    n94 = Insert Into Map(map in=w216, key=w217, value=w209) -> (map out=w214:map{T2, dbl})  [unwired: 2 out]
                    n95 = call "nanocal -- gradient descent.vi"("data"=w215, "action"=nanocal_--_gradient_descent_--_action."peek", "newton pars"=w211, "parameter keys IN"=w212, "parameter Map IN"=w214) -> ("goodness OUT"=w210:dbl)  [unwired: 2 in, 4 out]
                  }
                  n96 = Look In Map(map=w196, key=w195) -> (value=w194:dbl)  [unwired: 1 in, 1 out]
                  n97 = Look In Map(map=w202, key=w195) -> (value=w197:u32)  [unwired: 1 in, 1 out]
                  n98 = Look In Map(map=w201, key=w195) -> (value=w199:i32)  [unwired: 1 in, 1 out]
                  n99 = call "replace plot - plot ref - V2.vi"("Plot ref in"=w193, "Array X IN"=w206, "Array Y IN"=w207, "plot index"=w199, "cursor action"=cursor_action."write") -> ("Plot ref out"=w204:refnum<vi>)  [unwired: 11 in, 3 out]
                  n100 = call "replace cursor - plot ref - V2.vi"("Plot ref in"=w193, "new X"=w194, "cursor index"=w199, "cursor action"=cursor_action."write", "Color Box"=w197, "cursor state"=cursor_sate."colored") -> ()  [unwired: 10 in, 4 out]
                  n101 = call "replace plot - plot ref - V2.vi"("Plot ref in"=w204, "plot index"=w199, "cursor action"=cursor_action."set plot color", "Color Box"=w197) -> ()  [unwired: 12 in, 4 out]
                }
              }
              frame "2d plots " {
                n102 = for {
                  tunnel: w229 -> [w239]
                  tunnel: w228 -> [w238]
                  tunnel: w227 -> [w237] mode=indexing
                  tunnel: w226 -> [w236]
                  tunnel: w225 -> [w235]
                  shift-right: [w233] -> w222
                  shift-left: "{ " -> [w234]
                  tunnel: w220 -> [w232]
                  tunnel: w219 -> [w231]
                  tunnel: w218 -> [w230]
                  n103 = for {
                    tunnel: w236 -> [w247] mode=indexing
                    tunnel: w237 -> [w246]
                    tunnel: w239 -> [w260]
                    tunnel: w238 -> [w261]
                    tunnel: w235 -> [w259]
                    shift-right: [w256] -> w233
                    shift-left: w234 -> [w257]
                    tunnel: w232 -> [w244]
                    tunnel: w231 -> [w241]
                    tunnel: w230 -> [w240]
                    w250 = " ,     "
                    w255 = i16 12 ("precision (6)")
                    n104 = Insert Into Map(map in=w260, key=w261, value=w247) -> (map out=w258:map{T2, dbl})  [unwired: 2 out]
                    n105 = Number To Fractional String(number=w247, precision (6)=w255) -> (F-format string=w254:string)  [unwired: 2 in]
                    n106 = Number To Fractional String(number=w246, precision (6)=w255) -> (F-format string=w253:string)  [unwired: 2 in]
                    n107 = Insert Into Map(map in=w258, key=w259, value=w246) -> (map out=w245:map{T2, dbl})  [unwired: 2 out]
                    n108 = call "nanocal -- gradient descent.vi"("data"=w244, "action"=nanocal_--_gradient_descent_--_action."peek", "newton pars"=w240, "parameter keys IN"=w241, "parameter Map IN"=w245) -> ("goodness OUT"=w242:dbl)  [unwired: 2 in, 4 out]
                    n109 = Number To Fractional String(number=w242, precision (6)=w255) -> (F-format string=w252:string)  [unwired: 2 in]
                    n110 = Concatenate Strings(w257, "{    ", w254, w250, w253, w250, w252, " } , ", "\r") -> (w256:string)
                  }
                }
                n111 = Concatenate Strings(w222, " }   ") -> (→"2dplots":string)
              }
            }
          }
          frame "action: gradient step" {
            n112 = local write "newton is active"(TRUE ("newton is active")) -> ()
            n113 = call "nanocal -- publish -- freq scan V2.vi"("publisher action"=publisher_action."get") -> ("data"=w267:T34)  [unwired: 7 in, 3 out]
            n114 = call "nanocal -- gradient descent.vi"("data"=w267, "action"=nanocal_--_gradient_descent_--_action."init") -> ("goodness OUT"=w269:dbl)  [unwired: 5 in, 4 out]
            n115 = while {
              tunnel: w269 -> [_]
              tunnel: w265 -> [w289]
              tunnel: w266 -> [w279]
              tunnel: [w274] -> w263
              i -> [w275]
              stop <- w274 continue-if-true
              n116 = local read "newton is active"() -> (w290:bool)
              n117 = local read "factors"() -> (w293:cluster{"scaling":dbl, "what":T2}[])
              n118 = local read "newton parameters"() -> (w288:T3)
              n119 = Quotient & Remainder(x=w275, y="update rate") -> (x-y*floor(x/y)=w278:i32)  [unwired: 1 out]
              n120 = Less?(x=w275, y="total # steps") -> (x < y?=w276:bool)
              n121 = for {
                shift-right: [w313] -> w282
                shift-left: map{T2, dbl} {} ("Map IN") -> [w314]
                tunnel: w293 -> [w312] mode=indexing
                n122 = Unbundle(w312) -> ("scaling"=w310:dbl, "what"=w311:T2)
                n123 = Insert Into Map(map in=w314, key=w311, value=w310) -> (map out=w313:map{T2, dbl})  [unwired: 2 out]
              }
              n124 = local read "parameter map"() -> (w283:map{T2, dbl})
              n125 = And(x=w276, y=w290) -> (x .and. y?=w274:bool)
              n126 = case shown="0" w278 {
                tunnel: w279 -> [_ w297]
                frame 1, Default {
                }
                frame 0 {
                  n127 = Generate User Event(user event=w297, event data cluster="interface: update list from parameter map" ("event data")) -> (user event out=w296:refnum<user-event>)  [unwired: 2 in, 1 out]
                  n128 = Generate User Event(user event=w296, event data cluster="interface: update plot colors cursors" ("event data")) -> (user event out=w300:refnum<user-event>)  [unwired: 2 in, 1 out]
